vi "New.vi"(5 "Coordinates in":T1, 6 "Size in":dbl, 7 "Mass in":dbl, 9 "color in":u32(colorbox), 10 "Period (ms) in":dbl) -> (3 "Ball out":refnum<class "Ball.lvclass">)   [LabVIEW 2024, in "Ball.lvclass"]
doc: "MIT Licence\nCopyright (c) 2024 David Grollier"
uses:
  Ball.lvclass
  Type Def/Coordinates.ctl
  Type Def/Velocity.ctl
  Movable.lvclass/Movable.ctl
  Game Board Component.lvclass/Game Board Component.ctl
  Game Componants.lvclass/Game Componants.ctl
  Movable.lvclass
  Game Board Component.lvclass
  Game Componants.lvclass
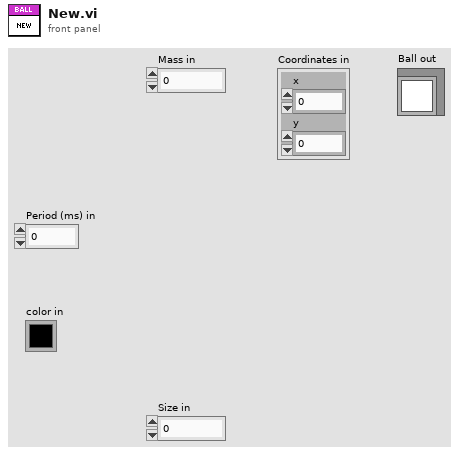
[diagram p1: front panel]
types:
  T1 = typedef "Coordinates.ctl" = cluster{"x":dbl, "y":dbl}
  T2 = typedef "Velocity.ctl" = cluster{"Vx":dbl, "Vy":dbl}
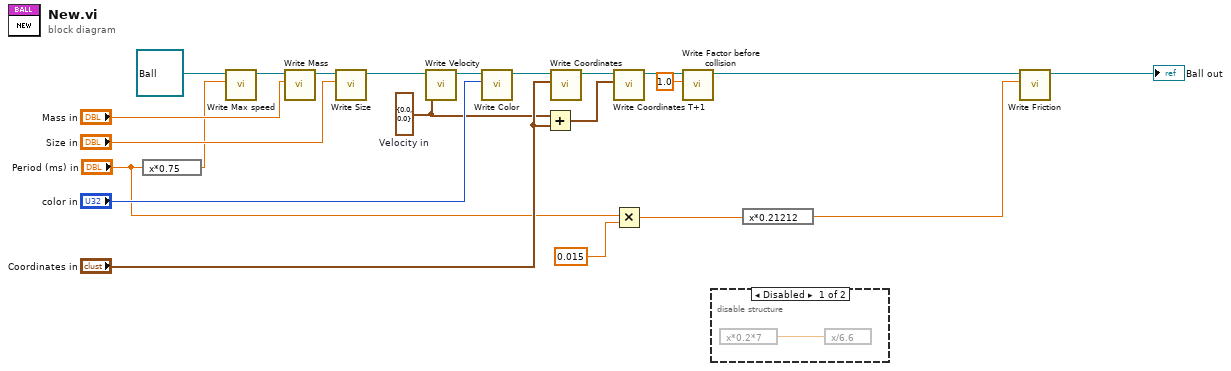
[diagram p0: block diagram]
diagram:
  w7 = T2 {"Vx"=0.0, "Vy"=0.0}  # Velocity in
  n1 = expression code="x*0.75"("Period (ms) in") -> (w6:dbl)
  n2 = call "Write Max speed.vi"("Max speed"=w6, "Movable in"=refnum<class "Ball.lvclass"> refnum ("Ball in")) -> ("Movable out"=w11:refnum<class "Ball.lvclass">)  [unwired: 9 in]
  n3 = call "Write Mass.vi"("Mass"="Mass in", "Movable in"=w11) -> ("Movable out"=w21:refnum<class "Ball.lvclass">)  [unwired: 9 in]
  n4 = call "Write Size.vi"("Size"="Size in", "Movable in"=w21) -> ("Movable out"=w20:refnum<class "Ball.lvclass">)  [unwired: 9 in]
  n5 = call "Write Velocity.vi"("Velocity"=w7, "Movable in"=w20) -> ("Movable out"=w17:refnum<class "Ball.lvclass">)  [unwired: 9 in]
  n6 = call "Write Color.vi"("color"="color in", "Game Board Component in"=w17) -> ("Game Board Component out"=w15:refnum<class "Ball.lvclass">)  [unwired: 9 in]
  n7 = Add(x=w7, y="Coordinates in") -> (x+y=w8:T2)
  n8 = call "Write Coordinates.vi"("Coordinates"="Coordinates in", "Game Componants in"=w15) -> ("Game Componants out"=w14:refnum<class "Ball.lvclass">)  [unwired: 9 in]
  n9 = call "Write Coordinates T+1.vi"("Coordinates"=w8, "Movable in"=w14) -> ("Movable out"=w10:refnum<class "Ball.lvclass">)  [unwired: 9 in]
  n10 = Multiply(x="Period (ms) in", y=0.015) -> (x*y=w2:dbl)
  n11 = call "Write Factor before collision.vi"("Factor before collision"=1.0, "Movable in"=w10) -> ("Movable out"=w12:refnum<class "Ball.lvclass">)  [unwired: 9 in]
  n12 = disable-structure shown="Disabled" {
    frame Disabled {
      n13 = expression code="x*0.2*7"() -> (w23:dbl)  [unwired: 1 in]
      n14 = expression code="x/6.6"(w23) -> ()  [unwired: 1 out]
    }
    frame Enabled {
    }
  }
  n15 = expression code="x*0.21212"(w2) -> (w3:dbl)
  n16 = call "Write Friction.vi"("Friction"=w3, "Movable in"=w12) -> ("Movable out"=→"Ball out":refnum<class "Ball.lvclass">)  [unwired: 9 in]
